vi "FTW-JSON-Object-SetElement-null.vi"(0 "JSON Object":refnum<data-value>, 5 "Key":string, 11 "error in":errorcluster) -> (4 "JSON Object out":refnum<data-value>, 15 "error out":errorcluster)   [LabVIEW 2015]
uses:
  core/FTW-JSON-Core-Structure.ctl
  error/FTW-ERR-ThrowError.vi
  error/FTW-ERR-CallChain.vi
  error/FTW-ERR-NoErrorConstant.vi
  string/FTW-STR-ReplaceWhitespace.vi
  string/FTW-STR-Array-Delimit.vi
panel:
  # "Inputs"
  # "Outputs"
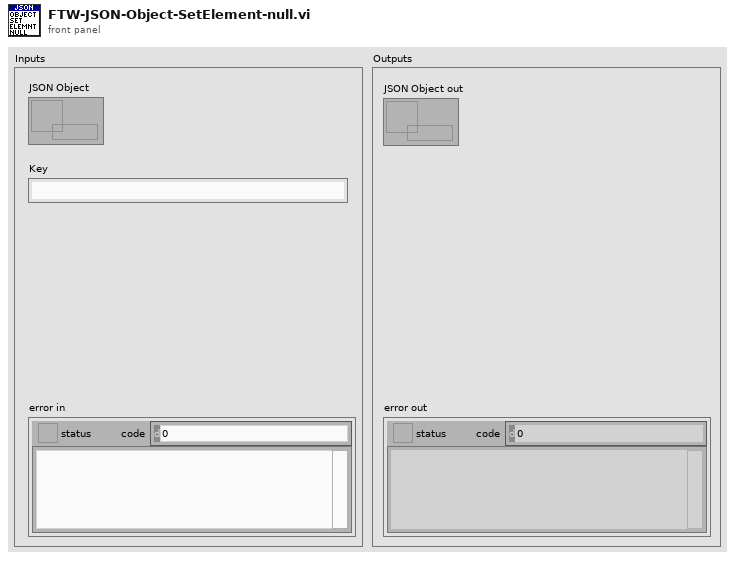
[diagram p1: front panel]
types:
  T1 = typedef "FTW-JSON-Core-Structure.ctl" = cluster{"JSON Object":i64, "Encoding Flags":i64, "Decoding Flags":i64}
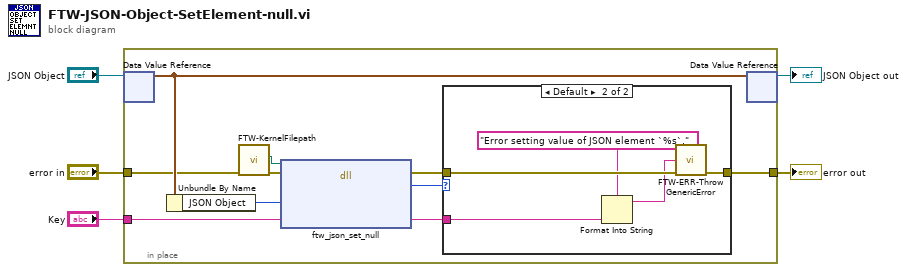
[diagram p0: block diagram]
diagram:
  n1 = in-place {
    in-place-border: "error in" -> [w8]
    in-place-border: [w9] -> w3
    in-place-border: "Key" -> [w15]
    n2 = in-place-dvr #1("JSON Object") -> (w14:T1)  [unwired: 1 out]
    n3 = Unbundle By Name(w14) -> ("JSON Object"=w13:i64)
    n4 = call "FTW-KernelFilepath.vi"("error in"=w8) -> ("error out"=w7:errorcluster, "Library Filepath"=w6:path)  [unwired: 8 in, 1 out]
    n5 = dll-call lib="?" fn="ftw_json_set_null"(path in=w6, error in=w7, "JSON Object Pointer"=w13, "Key"=w15) -> (error out=w11:errorcluster, "Return Value"=w12:i64, "Key"=w10:string)  [unwired: 2 in, 1 out]
    n6 = case shown="Default" w12 {
      tunnel: w11 -> [w16 w21]
      tunnel: w10 -> [_ w18]
      tunnel: [w16 w20] -> w9
      frame 0 {
      }
      frame Default {
        n7 = Format Into String(format string="Error setting value of JSON element `%s`.", w18) -> (resulting string=w17:string)  [unwired: 2 in, 1 out]
        n8 = call "FTW-ERR-ThrowGenericError.vi"("Error Message"=w17, "error in"=w21) -> ("error out"=w20:errorcluster)  [unwired: 13 in]
      }
    }
    n9 = in-place-dvr #1(w14) -> (→"JSON Object out":refnum<data-value>)  [unwired: 1 out]
  }
  "error out" <- w3
